vi "CalculateMicrostepFrequency.vi"(1 "div_i":i32, 2 "velocity":u16, 3 "clkdiv":i32) -> (0 "f_microstep":dbl)   [LabVIEW 2014, in "Sixpack - Driver.lvlib"]
doc: "This vi calculates the microstep frequency.\n(see Manual page 22)"
uses:
  Sixpack - Driver.lvlib
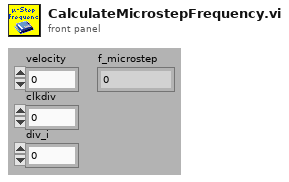
[diagram p1: front panel]
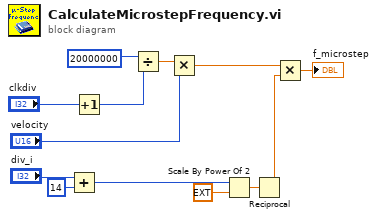
[diagram p0: block diagram]
diagram:
  n1 = Add(x="div_i", y=14) -> (x+y=w6:i32)
  n2 = Increment(x="clkdiv") -> (x+1=w11:i32)
  n3 = Divide(x=20000000, y=w11) -> (x/y=w10:dbl)
  n4 = Multiply(x=w10, y="velocity") -> (x*y=w3:dbl)
  n5 = Scale By Power Of 2(n=w6, x=ext 1.0) -> (x*2^n=w4:ext)
  n6 = Reciprocal(x=w4) -> (1/x=w2:ext)
  n7 = Multiply(x=w3, y=w2) -> (x*y=→"f_microstep":ext)
